vi "ReadSerialData.vi"() -> ()   [LabVIEW 2019]
uses:
  <vilib>/Instr/_visa.llb/VISA Configure Serial Port (Instr).vi
panel:
  in  "D":enum16{".5"}(ring)
  in  "I":enum16{"1"}(ring)
  in  "P":enum16{"25"}(ring)
  in  "cycle":enum16{"1000"}(ring)
  in  "Frequency":enum16{"1"}(ring)
  in  "Setpoint":enum16{"100"}(ring)
  in  "StartButton":bool
  out "Waveform Chart":cluster{u32, u32, u32, u32}(graph)
  in  "stop":bool
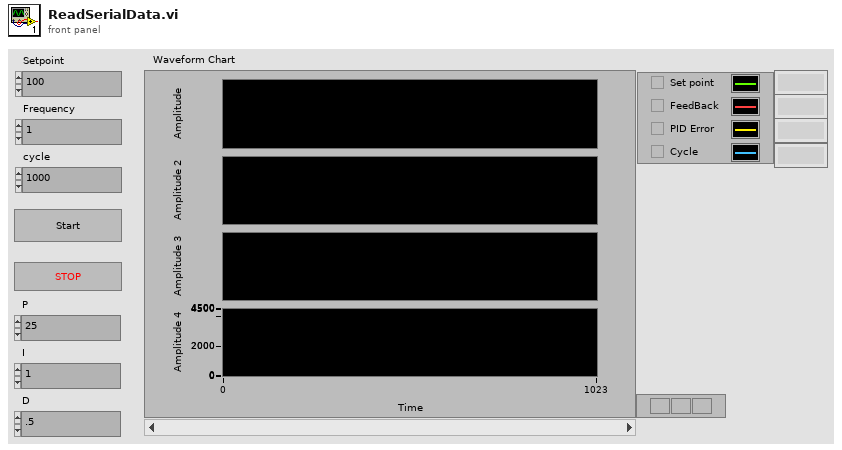
[diagram p1: front panel]
types:
  T1 = cluster{"SetPoint":u32, "FeedBack":u32, "PID":u32, "Cycle":u32}
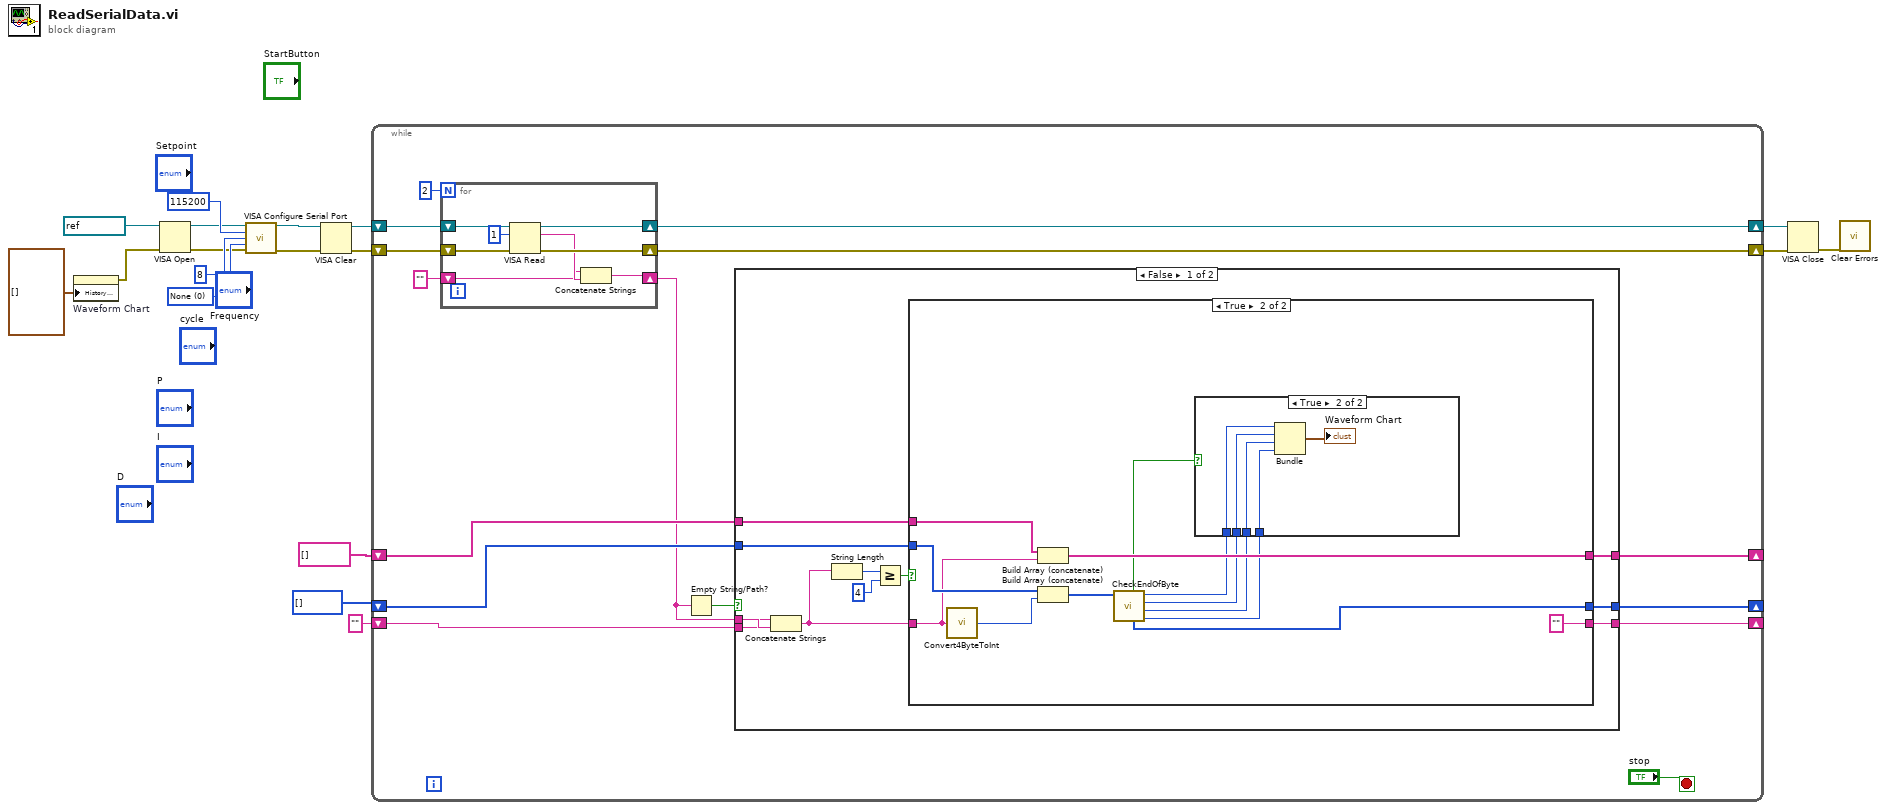
[diagram p0: block diagram]
diagram:
  w17 = u16 0 items=["None", "Odd", "Even", "Mark", "Space"] ("parity")
  n1 = property on="Waveform Chart" class="WFChart (strict)"("History Data"=cluster{u32, u32, u32, u32}[] []) -> (error out=w2:errorcluster)  [unwired: 2 in, 1 out]
  n2 = VISA Open(error in (no error)=w2, VISA resource name=refnum<visa-resource-name> "COM4") -> (VISA resource name=w15:refnum<visa-resource-name>, error out=w14:errorcluster)  [unwired: 3 in]
  n3 = call-poly "VISA Configure Serial Port"("VISA resource name"=w15, "baud rate (9600)"=u32 115200 ("baud rate"), "data bits (8)"=u16 8 ("data bits"), "parity (0:none)"=w17, "error in (no error)"=w14) -> ("VISA resource name out"=w8:refnum<visa-resource-name>, "error out"=w6:errorcluster)  [unwired: 4 in, 5 out]
  n4 = VISA Clear(VISA resource name=w8, error in (no error)=w6) -> (VISA resource name out=w7:refnum<visa-resource-name>, error out=w5:errorcluster)
  n5 = while {
    shift-right: [w30] -> _
    shift-left: "" -> [w29]
    shift-right: [w28] -> w11
    shift-left: w5 -> [w32]
    shift-right: [w27] -> w10
    shift-left: w7 -> [w33]
    shift-right: [w24] -> _
    shift-left: u32[] [] -> [w25]
    shift-right: [w22] -> _
    shift-left: string[] [] -> [w23]
    stop <- "stop" stop-if-true
    n6 = for {
      N: 2 -> [_]
      shift-right: [w37] -> w27
      shift-left: w33 -> [w41]
      shift-right: [w38] -> w28
      shift-left: w32 -> [w40]
      shift-right: [w34] -> w19
      shift-left: "" ("read buffer") -> [w35]
      n7 = VISA Read(VISA resource name=w41, byte count=u32 1, error in (no error)=w40) -> (VISA resource name out=w37:refnum<visa-resource-name>, read buffer=w36:string, error out=w38:errorcluster)  [unwired: 1 out]
      n8 = Concatenate Strings(w35, w36) -> (w34:string)
    }
    n9 = Empty String/Path?(string/path=w19) -> (empty?=w26:bool)
    n10 = case shown="False" w26 {
      tunnel: w19 -> [w52 _]
      tunnel: [w44 w76] -> w30
      tunnel: w29 -> [w51 w76]
      tunnel: w25 -> [w46 w75]
      tunnel: [w45 w75] -> w24
      tunnel: [w43 w74] -> w22
      tunnel: w23 -> [w42 w74]
      frame False {
        n11 = Concatenate Strings(w51, w52) -> (w47:string)
        n12 = String Length(string=w47) -> (length=w50:i32)
        n13 = Greater Or Equal?(x=w50, y=4) -> (x >= y?=w48:bool)
        n14 = case shown="True" w48 {
          tunnel: w47 -> [w54 w65]
          tunnel: w46 -> [w55 w68]
          tunnel: [w55 w61] -> w45
          tunnel: [w54 ""] -> w44
          tunnel: [w53 w64] -> w43
          tunnel: w42 -> [w53 w63]
          frame False {
          }
          frame True {
            n15 = call "Convert4ByteToInt.vi"("Input"=w65) -> ("Output"=w66:u32)
            n16 = Build Array (concatenate)(w63, w65) -> (w64:string[])
            n17 = Build Array (concatenate)(w68, w66) -> (w62:u32[])
            n18 = call "CheckEndOfByte.vi"("Input"=w62) -> ("Cycle"=w57:u32, "PID"=w58:u32, "FeedBack"=w59:u32, "SetPoint"=w60:u32, "RemainingData"=w61:u32[], "Plot?"=w56:bool)  [unwired: 5 in]
            n19 = case shown="True" w56 {
              tunnel: w60 -> [_ w73]
              tunnel: w59 -> [_ w72]
              tunnel: w58 -> [_ w71]
              tunnel: w57 -> [_ w70]
              frame False {
              }
              frame True {
                n20 = Bundle("SetPoint"=w73, "FeedBack"=w72, "PID"=w71, "Cycle"=w70) -> (→"Waveform Chart":T1)  [unwired: 1 in]
              }
            }
          }
        }
      }
      frame True {
      }
    }
  }
  n21 = VISA Close(VISA resource name=w10, error in (no error)=w11) -> (error out=w9:errorcluster)
  n22 = call <vilib>:"Clear Errors.vi"("error in (no error)"=w9) -> ()  [unwired: 5 in, 2 out]
